vi "pass2color.vi"(1 "pass?":bool) -> (0 "color":u32)   [LabVIEW 2024]
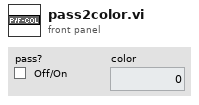
[diagram p1: front panel]
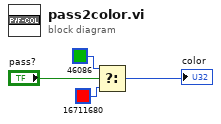
[diagram p0: block diagram]
diagram:
  n1 = Select(t=u32 46086 ("Numeric Text.Text Colors:Text Color"), s="pass?", f=u32 16711680 ("Numeric Text.Text Colors:Text Color")) -> (s? t:f=→"color":u32)
